vi "DB Get Current Users.vi"(8 "error in (no error)":errorcluster) -> (0 "error out":errorcluster, 2 "Result (Rows or Columns)":string[](array[string]))   [LabVIEW 2019, in "Control Experiment.lvclass"]
uses:
  Control Experiment.lvclass
  <vilib>/JDP Science/PostgreSQL Library/Connection/Execute Command (1D string results).vi
  <vilib>/JDP Science/PostgreSQL Library/Connection/Execute Command (Result).vi
  <vilib>/JDP Science/PostgreSQL Library/Result/Get all results as 1D strings array.vi
  <vilib>/JDP Science/PostgreSQL Library/Result/Get Column Headers.vi
  <vilib>/JDP Science/PostgreSQL Library/Result/Clear.vi
  <vilib>/JDP Science/PostgreSQL Library/Connection/PQ Connection.lvclass
  <userlib>/LevyLab/LV-Data/LV-Data.PG/PGPASS/PGPASS.lvlib
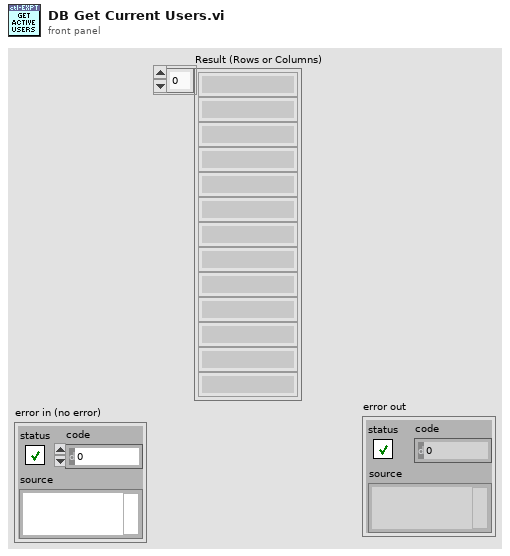
[diagram p1: front panel]
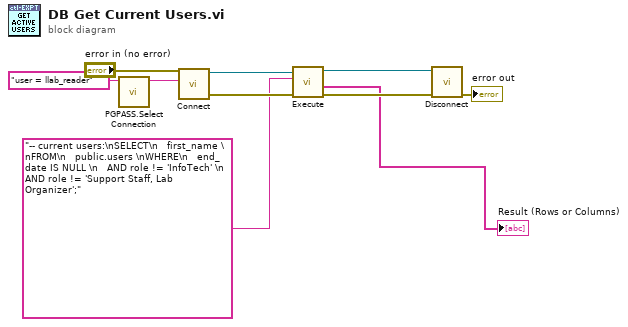
[diagram p0: block diagram]
diagram:
  n1 = call <userlib>:"PGPASS.Select Connection.vi"("search string"="user = llab_reader") -> ("connection string"=w10:string)  [unwired: 9 in, 1 out]
  n2 = call <vilib>:"Connect.vi"("error in (no error)"="error in (no error)", "Connection Strings"=w10) -> ("error out"=w7:errorcluster, "PQ Connection"=w8:refnum<class "PQ Connection.lvclass">)  [unwired: 8 in]
  n3 = call-poly <vilib>:"Execute.vi"("error in (no error)"=w7, "SQL"="-- current users:\nSELECT\n   first_name \nFROM\n   public.users \nWHERE\n   end_date IS NULL \n   AND role != 'InfoTech' \n   AND role != 'Support Staff, Lab Organizer';" ("Address"), "PQ Connection in"=w8) -> ("error out"=w4:errorcluster, "Result (Rows or Columns)"=→"Result (Rows or Columns)":string[], "PQ Connection out"=w5:refnum<class "PQ Connection.lvclass">)  [unwired: 4 in, 2 out]
  n4 = call <vilib>:"Disconnect.vi"("error in (no error)"=w4, "PQ Connection in"=w5) -> ("error out"=→"error out":errorcluster)  [unwired: 9 in]
